vi "Histogram.vi"(8 "error in":errorcluster, 11 "Refnum in":T2) -> (0 "error out":errorcluster, 3 "Histogram OUT":T1)   [LabVIEW 2013]
uses:
  <vilib>/vision/Image Controls.llb/IMAQ Image.ctl
  <vilib>/vision/NI_Vision_Development_Module.lvlib
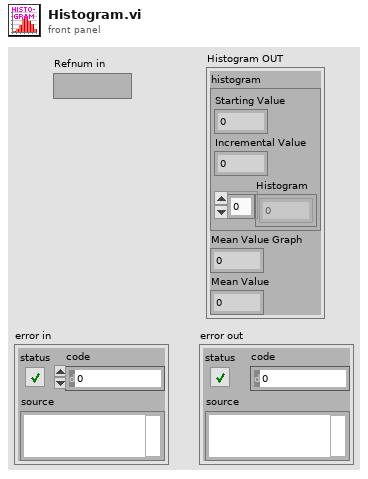
[diagram p1: front panel]
types:
  T1 = cluster{"histogram":cluster{"Starting Value":sgl, "Incremental Value":sgl, "Histogram":u32[]}, "Mean Value Graph":sgl, "Mean Value":sgl}
  T2 = typedef "IMAQ Image.ctl" = refnum<image>
  T3 = cluster{"Starting Value":sgl, "Incremental Value":sgl, "Histogram":u32[]}
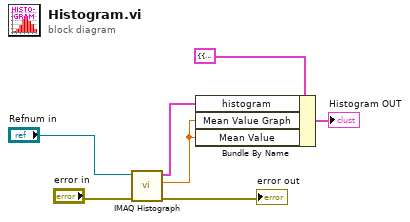
[diagram p0: block diagram]
diagram:
  n1 = call "IMAQ Histograph"("error in (no error)"="error in", "Image"="Refnum in") -> ("error out"=→"error out":errorcluster, "Mean Value"=w1:sgl, "Histogram Graph"=w2:T3)  [unwired: 6 in, 1 out]
  n2 = Bundle By Name(cluster=T1 {"histogram"={"Starting Value"=0.0, "Incremental Value"=0.0, "Histogram"=[]}, "Mean Value Graph"=0.0, "Mean Value"=0.0} ("Histogram OUT"), "histogram"=w2, "Mean Value Graph"=w1, "Mean Value"=w1) -> (→"Histogram OUT":T1)
